vi "Demo.vi"() -> ()   [LabVIEW 2018]
uses:
  S7-1500Lib/SPSCom_S1500/S1500_test_S7Com_HexByteArray.ctl
  S7-1500Lib/SPSCom_S1500/S1500_S7Com_HexByte.ctl
  S7-1500Lib/SPSCom_S1500/S1500_S7Com_RW_CMD.ctl
  S7-1500Lib/SPSCom_S1500/S1500_S7Com_Address_Area.ctl
  S7-1500Lib/SPSCom_S1500/S1500_S7Com_Start_Add.ctl
  S7-1500Lib/SPSCom_S1500/S1500_S7Com_Transport_Size.ctl
  S7-1500Lib/SPSCom_S1500/S1500_S7Com_Function.ctl
  S7-1500Lib/SPSCom_S1500/S1500_S7Com_Data_Array.ctl
panel:
  in  "WriteToPLC":bool
  in  "Write_Data":T1=[1, 1, 1, 1]
  in  "Write_CMD":T2={"Read Length"=1, "Data Block #"=2, "S7_Add_Area"=132, "Start Address"=0, "S7_Transport_Size"=5, "S7_Function"=5, "IP-Address"=""} {"S7_Function" items=["Read"=4, "Write"=5]; "S7_Transport_Size" items=["BIT"=1, "BYTE"=2, "CHAR"=3, "WORD"=4, "INT"=5, "DWORD"=6, "DINT"=7, "REAL"=8]; "S7_Add_Area" items=["P Area"=128, "I Area"=129, "O Area"=130, "M Area"=131, "DB Area"=132, "Counter"=40, "Timer"=41]}
  out "ReadTime":u32
  out "WriteTime":u32
  out "WriteError?":bool
  out "ReadError?":bool
  out "Read_Data":T1=[1, 1, 257, 2, 3404, 0, 3404, 17748, -16384, 0, 0, 0, 0, 0, 0, 0, 0, 0, 0, 0, 0, 0, 0, 0, 0, 0, 0, 0, 0, 0, 0, 0, 0, 0, 0, 0, 0, 0, 0, 0, 0, 0, 0, 0, 0, 0, 0, 0, 0, 0, 0, 0, 0, 0, 0, 0, 0, 0, 0, 0, 0, 0, 0, 0, 0, 0, 0, 0, 0, 0, 0, 0, 0, 0, 0, 0, 0, 0, 0, 0, 0, 0, 0, 0, 0, 0, 0, 0, 0, 0, 0, 0, 0, 0, 0, 0, 0, 0, 0, 0, 0, 0, 0, 0, 0, 0, 0, 0, 0, 0, 0, 0, 0, 0, 0]
  in  "Read_CMD":T2={"Read Length"=115, "Data Block #"=2, "S7_Add_Area"=132, "Start Address"=0, "S7_Transport_Size"=5, "S7_Function"=4, "IP-Address"=""} {"S7_Function" items=["Read"=4, "Write"=5]; "S7_Transport_Size" items=["BIT"=1, "BYTE"=2, "CHAR"=3, "WORD"=4, "INT"=5, "DWORD"=6, "DINT"=7, "REAL"=8]; "S7_Add_Area" items=["P Area"=128, "I Area"=129, "O Area"=130, "M Area"=131, "DB Area"=132, "Counter"=40, "Timer"=41]}
  out "PDU Response":T7=[50, 3, 0, 0, 2, 0, 0, 8, 0, 0, 0, 0, 240, 0, 0, 1, 0, 1, 1, 224] format="X%02x"
  out "Error":bool
  in  "remote port":u16=102
  in  "remote address":string="192.168.6.100"
  out "error out":errorcluster caption="错误输出"
  in  "error in (no error)":errorcluster caption="错误输入（无错误）"
  in  "停止":bool
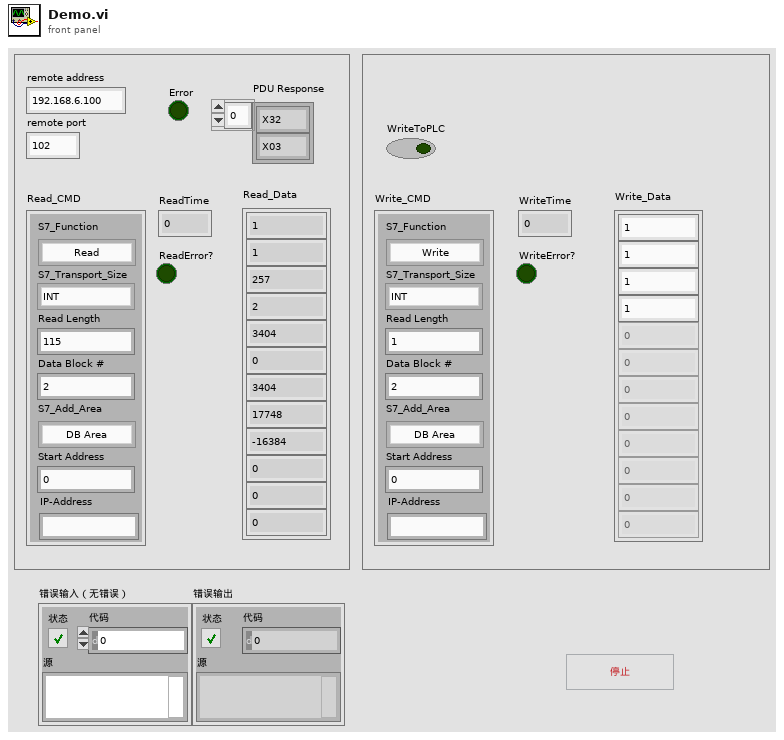
[diagram p1: front panel]
types:
  T1 = typedef "S1500_S7Com_Data_Array.ctl" = i32[]
  T2 = typedef "S1500_S7Com_RW_CMD.ctl" = cluster{"Read Length":u16, "Data Block #":u16, "S7_Add_Area":T3, "Start Address":T4, "S7_Transport_Size":T5, "S7_Function":T6, "IP-Address":string}
  T3 = typedef "S1500_S7Com_Address_Area.ctl" = u8
  T4 = typedef "S1500_S7Com_Start_Add.ctl" = u16
  T5 = typedef "S1500_S7Com_Transport_Size.ctl" = u8
  T6 = typedef "S1500_S7Com_Function.ctl" = u8
  T7 = typedef "S1500_test_S7Com_HexByteArray.ctl" = T8[]
  T8 = typedef "S1500_S7Com_HexByte.ctl" = u8
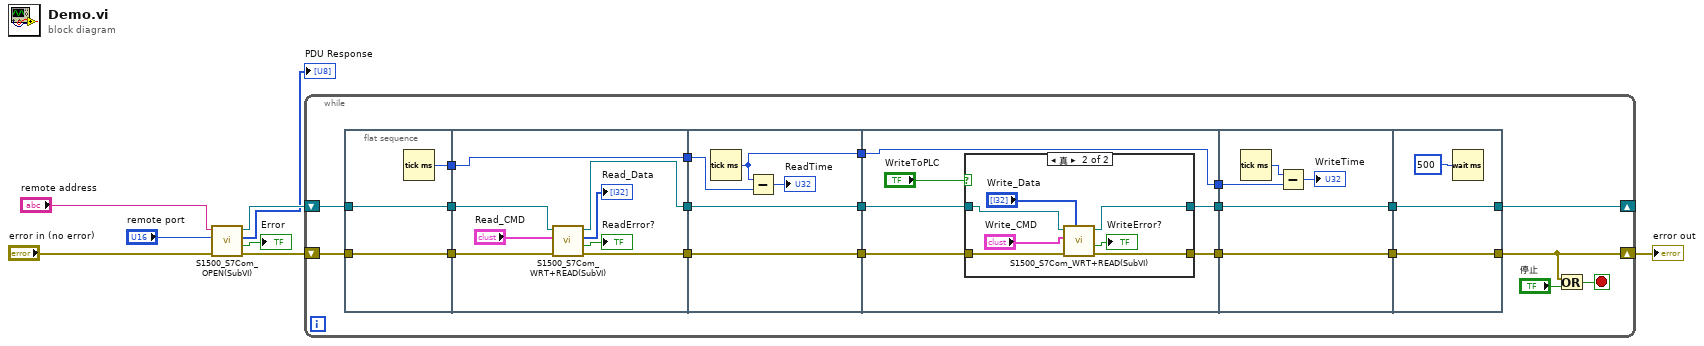
[diagram p0: block diagram]
diagram:
  n1 = call "S1500_S7Com_OPEN(SubVI).vi"("remote address"="remote address", "remote port"="remote port", "error in (no error)"="error in (no error)") -> ("connection ID out"=w7:refnum<k5>, "PDU Response"=→"PDU Response":T7, "Error"=→"Error":bool, "error out"=w2:errorcluster)  [unwired: 1 in, 1 out]
  n2 = while {
    shift-right: [w12] -> _
    shift-left: w7 -> [w23]
    shift-right: [w9] -> w8
    shift-left: w2 -> [w21]
    stop <- w15 stop-if-true
    n3 = flat-sequence {
      tunnel: [w31] -> w26
      tunnel: [w30] -> w24
      tunnel: w23 -> [w30]
      tunnel: [w29] -> w22
      tunnel: w21 -> [w29]
      tunnel: w26 -> [w39]
      tunnel: [w39] -> w25
      tunnel: w24 -> [w38]
      tunnel: w22 -> [w37]
      tunnel: [w35] -> w20
      tunnel: [w32] -> w18
      tunnel: [w44] -> w28
      tunnel: w25 -> [w43]
      tunnel: w20 -> [w42]
      tunnel: [w42] -> w19
      tunnel: w18 -> [w41]
      tunnel: [w41] -> w17
      tunnel: w28 -> [w50]
      tunnel: [w50] -> w27
      tunnel: w19 -> [w49]
      tunnel: w17 -> [w48]
      tunnel: [w47] -> w16
      tunnel: [w46] -> w10
      tunnel: w27 -> [w63]
      tunnel: w16 -> [w62]
      tunnel: [w62] -> w13
      tunnel: [w60] -> w11
      tunnel: w10 -> [w60]
      tunnel: [w67] -> w9
      tunnel: w13 -> [w67]
      tunnel: [w65] -> w12
      tunnel: w11 -> [w65]
      frame #0 {
        n4 = Tick Count (ms)() -> (millisecond timer value=w31:u32)
      }
      frame #1 {
        n5 = call "S1500_S7Com_WRT+READ(SubVI).vi"("error in"=w37, "RW_CMD"="Read_CMD", "connection ID in"=w38) -> ("error out"=w32:errorcluster, "Error"=→"ReadError?":bool, "Read_Data"=→"Read_Data":T1, "connection ID out"=w35:refnum<k5>)  [unwired: 2 in]
      }
      frame #2 {
        n6 = Tick Count (ms)() -> (millisecond timer value=w44:u32)
        n7 = Subtract(x=w44, y=w43) -> (x-y=→"ReadTime":u32)
      }
      frame #3 {
        n8 = case shown="真" "WriteToPLC" {
          tunnel: w49 -> [w52 w59]
          tunnel: w48 -> [w51 w57]
          tunnel: [w51 w56] -> w47
          tunnel: [w52 w54] -> w46
          frame False {
          }
          frame True {
            n9 = call "S1500_S7Com_WRT+READ(SubVI).vi"("Write_Data"="Write_Data", "error in"=w57, "RW_CMD"="Write_CMD", "connection ID in"=w59) -> ("error out"=w56:errorcluster, "Error"=→"WriteError?":bool, "connection ID out"=w54:refnum<k5>)  [unwired: 1 in, 1 out]
          }
        }
      }
      frame #4 {
        n10 = Tick Count (ms)() -> (millisecond timer value=w64:u32)
        n11 = Subtract(x=w64, y=w63) -> (x-y=→"WriteTime":u32)
      }
      frame #5 {
        n12 = Wait (ms)(milliseconds to wait=u32 500 ("等待时间（毫秒）")) -> ()  [unwired: 1 out]
      }
    }
    n13 = Or(x=w9, y="停止") -> (x .or. y?=w15:bool)
  }
  "error out" <- w8
